vi "SUT.vi"() -> (2 "String 2":string, 3 "String":string)   [LabVIEW 2020]
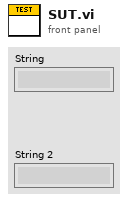
[diagram p1: front panel]
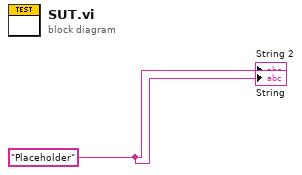
[diagram p0: block diagram]
diagram:
  w1 = "Placeholder"
  "String" <- w1
  "String 2" <- w1
